vi "Stop.vi"(8 "error in":errorcluster, 11 "CAN Task in":refnum<class "CANopen Task Actor.lvclass">) -> (0 "error out":errorcluster, 3 "CAN Task out":refnum<class "CANopen Task Actor.lvclass">)   [LabVIEW 2024, in "CANopen Task Actor.lvlib" / "CANopen Task Actor.lvclass"]
uses:
  CANopen Task Actor.lvclass
  CANopen Task Actor.lvclass/CANopen Task Actor.ctl
  <vilib>/ActorFramework/Time-Delayed Send Message/Time-Delay Override Options.ctl
  CANopen.lvclass
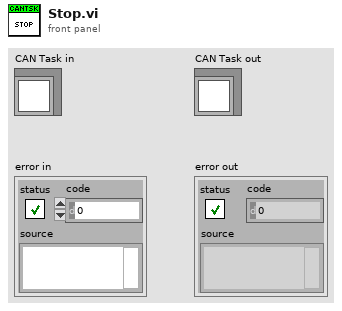
[diagram p1: front panel]
types:
  T1 = typedef "Time-Delay Override Options.ctl" = enum16{"Send next copy now", "Skip next scheduled copy", "Send next copy now and stop all further copies", "Stop all further copies"}
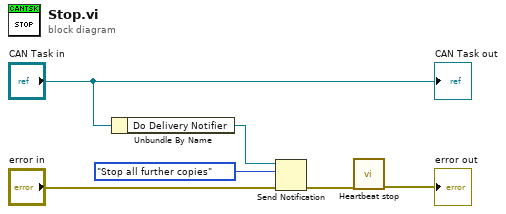
[diagram p0: block diagram]
diagram:
  n1 = Unbundle By Name("CAN Task in") -> ("Do Delivery Notifier"=w6:refnum<notifier>)
  n2 = Send Notification(notification=Time-Delay_Override_Options."Stop all further copies" ("Time Delay Override Options"), notifier=w6, error in (no error)="error in") -> (error out=w2:errorcluster)  [unwired: 1 out]
  n3 = call "Heartbeat stop.vi"("error in"=w2) -> ("error out"=→"error out":errorcluster)  [unwired: 2 in, 4 out]
  "CAN Task out" <- "CAN Task in"
